vi "Convert to String.vi"(10 "Byte Array":u8[](array[numeric]), 11 "number of objects":u8) -> (3 "Objects":T1[](array[typedef]) {"Object ID" format="%x"})   [LabVIEW 2013, in "Modbus Library - Advance.lvlib" / "Master Function Definition.lvclass"]
uses:
  Master Function Definition.lvclass
  Data Model/Identification Parameters.ctl
  Data Model/Device Data Model.lvclass
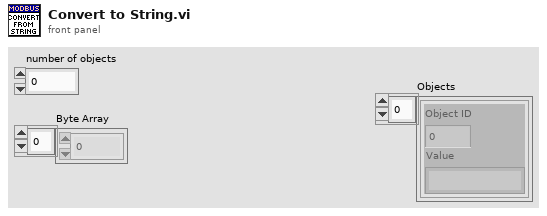
[diagram p1: front panel]
types:
  T1 = typedef "Modbus Library - Advance.lvlib/Device Data Model.lvclass/Identification Parameters.ctl" = cluster{"Object ID":u8, "Value":string}
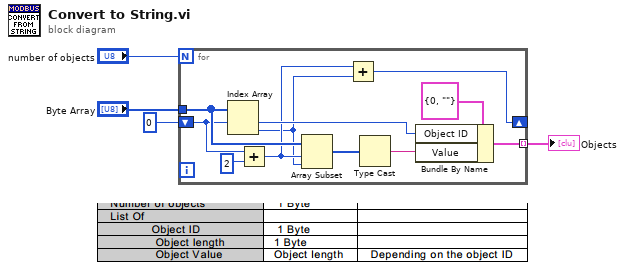
[diagram p0: block diagram]
diagram:
  n1 = for {
    N: "number of objects" -> [_]
    shift-right: [w6] -> _
    shift-left: 0 -> [w9]
    tunnel: [w14] -> w1 mode=indexing
    tunnel: "Byte Array" -> [w11]
    n2 = Index Array(array=w11, index #1=w9) -> (element #1=w12:u8, element #2=w5:u8)  [unwired: 1 in]
    n3 = Add(x=w9, y=2) -> (x+y=w7:i32)
    n4 = Array Subset(array=w11, index=w7, length=w5) -> (w10:u8[])
    n5 = Add(x=w7, y=w5) -> (x+y=w6:i32)
    n6 = Type Cast(x=w10) -> (*(type *) &x=w13:string)  [unwired: 1 in]
    n7 = Bundle By Name(cluster=T1 {"Object ID"=0, "Value"=""} ("Cluster"), "Object ID"=w12, "Value"=w13) -> (w14:T1)
  }
  "Objects" <- w1
